vi "MeasureHeights.vi"() -> ()   [LabVIEW 2019]
uses:
  <vilib>/Math Plots/3D Math Plots/3D Surface/3D Surface XCtrl/3D Surface.xctl
  <vilib>/Math Plots/3D Math Plots/3D Surface/3D Surface Datatype/Public/Plot Helper (Matrix).vi
  <vilib>/Math Plots/3D Math Plots/3D Surface/3D Surface Datatype/3D Surface Datatype.lvclass
panel:
  in  "OutFile":path=path "C:/Users/TTUHEP/Documents/LabVIEW/Data/AssemblyIO_logs/Ouput/DistanceSenOutData.txt"
  out "3D Surface":refnum<class "3D Plot Datatype.lvclass">[](xcontrol)
  out "sd":dbl[](array[numeric])
  out "Dist":dbl[](array[numeric])
  in  "NumberLines":i32
  in  "Locations":path=path "C:/Users/TTUHEP/Documents/LabVIEW/Data/AssemblyIO_logs/Inputs/DistSensMeasureLocations.txt"
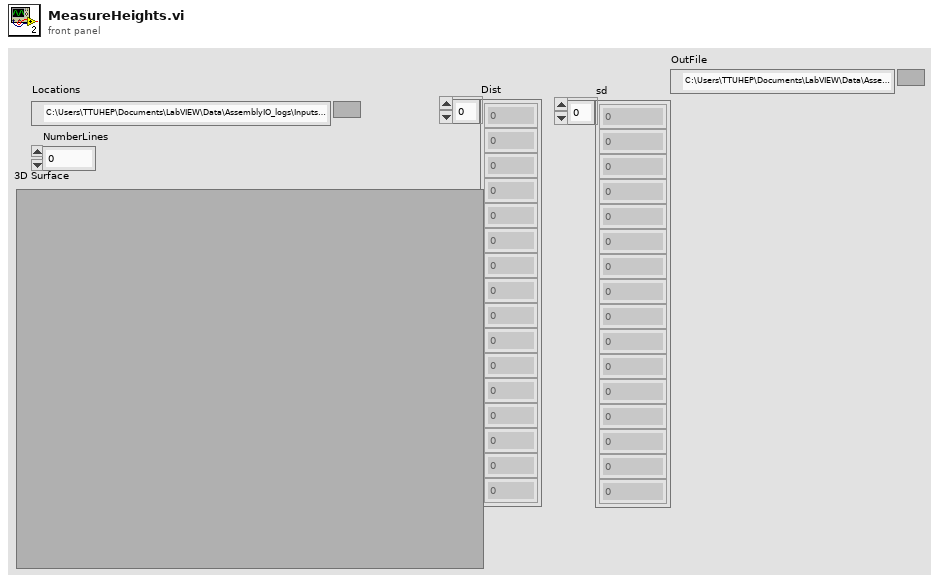
[diagram p1: front panel]
types:
  T1 = enum16{"open", "replace", "create", "open or create", "replace or create", "replace or create with confirmation"}
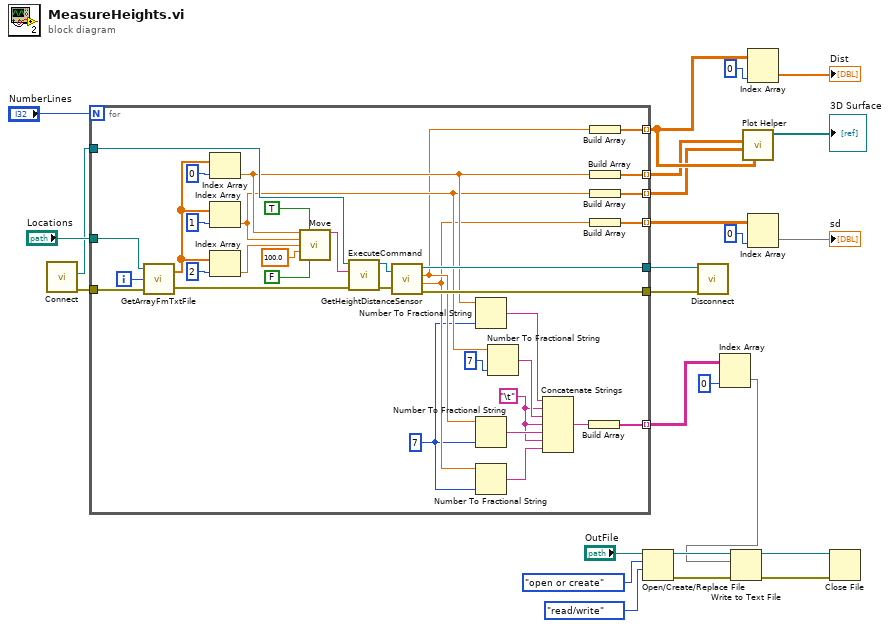
[diagram p0: block diagram]
diagram:
  n1 = call "Connect.vi"() -> ("error out"=w24:errorcluster, "controller"=w18:refnum<k24>)  [unwired: 10 in]
  n2 = for {
    N: "NumberLines" -> [_]
    tunnel: "Locations" -> [w51]
    tunnel: w24 -> [w50]
    tunnel: [w46] -> w13 mode=indexing
    tunnel: [w45] -> w21 mode=indexing
    tunnel: [w44] -> w20
    tunnel: [w43] -> w19
    tunnel: w18 -> [w42]
    tunnel: [w40] -> w12 mode=indexing
    tunnel: [w39] -> w11 mode=indexing
    tunnel: [w26] -> w3 mode=indexing
    i -> [w41]
    w31 = "\t"
    w29 = i16 7 ("precision (6)")
    n3 = call "GetArrayFmTxtFile.vi"("error in"=w50, "LineNo."=w41, "TextFile"=w51) -> ("error out"=w53:errorcluster, "Array"=w57:dbl[])
    n4 = Index Array(array=w57, index=0) -> (element=w38:dbl)
    n5 = Index Array(array=w57, index=1) -> (element=w36:dbl)
    n6 = Index Array(array=w57, index=2) -> (element=w52:dbl)
    n7 = call "Move.vi"("X"=w38, "Absolute"=TRUE, "Y"=w36, "Z"=w52, "SpeedXY (mm/s)"=100.0, "Move Z first"=FALSE) -> ("Position Gcode"=w54:string)  [unwired: 9 in]
    n8 = call "ExecuteCommand.vi"("error in (no error)"=w53, "Command Code"=w54, "controller in"=w42) -> ("error out"=w48:errorcluster, "controller out"=w47:refnum<k24>)  [unwired: 6 in, 1 out]
    n9 = call "GetHeightDistanceSensor.vi"("controller in"=w47, "error in (no error)"=w48) -> ("controller out"=w43:refnum<k24>, "MeanHeight(mm)"=w33:dbl, "SDofHeight(mm)"=w30:dbl, "error out"=w44:errorcluster)
    n10 = Number To Fractional String(number=w38, precision (6)=w29) -> (F-format string=w35:string)  [unwired: 2 in]
    n11 = Number To Fractional String(number=w33, precision (6)=w29) -> (F-format string=w32:string)  [unwired: 2 in]
    n12 = Number To Fractional String(number=w30, precision (6)=w29) -> (F-format string=w28:string)  [unwired: 2 in]
    n13 = Number To Fractional String(number=w36, precision (6)=i16 7) -> (F-format string=w34:string)  [unwired: 2 in]
    n14 = Concatenate Strings(w35, w31, w34, w31, w32, w31, w28) -> (w27:string)
    n15 = Build Array(w27) -> (w26:string[])
    n16 = Build Array(w33) -> (w46:dbl[])
    n17 = Build Array(w38) -> (w40:dbl[])
    n18 = Build Array(w36) -> (w39:dbl[])
    n19 = Build Array(w30) -> (w45:dbl[])
  }
  n20 = Open/Create/Replace File(file path (use dialog)="OutFile", operation (0:open)=T1."open or create", access (0:read/write)=enum16{"read/write", "read-only", "write-only"}."read/write") -> (refnum out=w10:refnum<file>, error out=w7:errorcluster)  [unwired: 3 in, 1 out]
  n21 = call "Disconnect.vi"("error in (no error)"=w20, "controller"=w19) -> ()  [unwired: 9 in, 1 out]
  n22 = Index Array(array=w3, index (col)=0 ("disabled index (col)")) -> (element=w1:string[])  [unwired: 1 in]
  n23 = Write to Text File(file (use dialog)=w10, text=w1, error in=w7) -> (refnum out=w5:refnum<file>, error out=w6:errorcluster)  [unwired: 1 in, 1 out]
  n24 = call-poly <vilib>:"Plot Helper.vi"("z matrix"=w13, "y matrix"=w11, "x matrix"=w12) -> ("3D Plot lvclass Array out"=→"3D Surface":refnum<class "3D Plot Datatype.lvclass">[])  [unwired: 3 in, 5 out]
  n25 = Index Array(array=w13, index (col)=0 ("disabled index (col)")) -> (element=→"Dist":dbl[])  [unwired: 1 in]
  n26 = Index Array(array=w21, index (col)=0 ("disabled index (col)")) -> (element=→"sd":dbl[])  [unwired: 1 in]
  n27 = Close File(refnum=w5, error in=w6) -> ()  [unwired: 2 out]
